vi "Read Stderr.vi"(8 "Error In":errorcluster, 10 "Max Data Length":i32=1024, 11 "Channel In":refnum<class "Channel.lvclass">) -> (0 "Error Out":errorcluster, 1 "End-of-File?":bool, 2 "Data":u8[](array[numeric]), 3 "Channel Out":refnum<class "Channel.lvclass">)   [LabVIEW 2018, in "Toolkit.lvlib" / "Channel.lvclass"]
uses:
  Channel.lvclass
  Channel.lvclass/Channel.ctl
  Session/Session.lvclass/Session.ctl
  SSH/SSH.lvclass/SSH.ctl
  Session/Session.lvclass
  Toolkit.lvlib
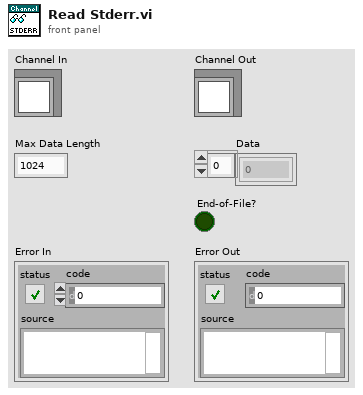
[diagram p1: front panel]
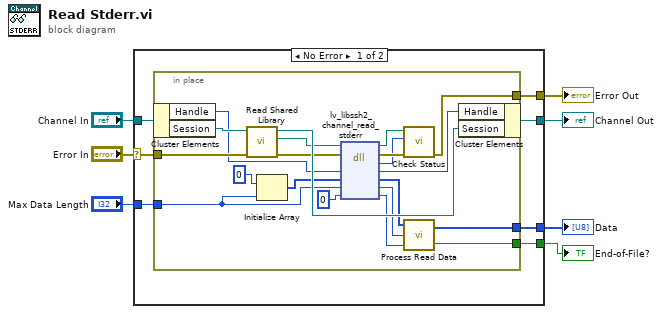
[diagram p0: block diagram]
diagram:
  n1 = case shown="No Error" "Error In" {
    selector: "Error In" -> [w12 w36]
    tunnel: [w11 w36] -> w6
    tunnel: "Channel In" -> [w14 w35]
    tunnel: [w13 w35] -> w4
    tunnel: "Max Data Length" -> [w10 _]
    tunnel: [w9 _] -> w2
    tunnel: [w8 _] -> w1
    frame No Error {
      n2 = in-place {
        in-place-border: w12 -> [w30]
        in-place-border: [w26] -> w11
        in-place-border: w10 -> [w20]
        in-place-border: [w18] -> w9
        in-place-border: [w15] -> w8
        n3 = in-place-cluster #1(w14) -> ("Handle"=w25:u64, "Session"=w34:refnum<class "Session.lvclass">)
        n4 = call "Read Shared Library.vi"("Error In"=w30, "Session In"=w34) -> ("Erorr Out"=w31:errorcluster, "libssh2lv Shared Library"=w32:path, "Session Out"=w33:refnum<class "Session.lvclass">)  [unwired: 7 in]
        n5 = Initialize Array(u8 0, w20) -> (w23:u8[])
        n6 = dll-call lib="libssh2lv.*" fn="lv_libssh2_channel_read_stderr"(path in=w32, error in=w31, "handle"=w25, "buffer"=w23, "buffer_len"=w20, "byte_count"=u64 0) -> (path out=w28:path, error out=w29:errorcluster, "status"=w27:i32, "handle"=w24:u64, "buffer"=w19:u8[], "buffer_len"=w17:u64, "byte_count"=w16:u64)  [unwired: 1 in]
        n7 = call "Check Status.vi"("Error In"=w29, "Status"=w27, "lv-libssh2 Shared Library In"=w28) -> ("Error Out"=w26:errorcluster)  [unwired: 7 in, 1 out]
        n8 = call "Process Read Data.vi"("Bytes Read Count"=w16, "Max Data Length"=w17, "Data In"=w19) -> ("End-of-File?"=w15:bool, "Data Out"=w18:u8[])
        n9 = in-place-cluster #1("Handle"=w24, "Session"=w33) -> (w13:refnum<class "Channel.lvclass">)
      }
    }
    frame Error {
    }
  }
  "Error Out" <- w6
  "Channel Out" <- w4
  "End-of-File?" <- w1
  "Data" <- w2
